vi "add-spectrum-eventSD.vi"(1 "cluster in":T1={"Kinetics"=[], "Spectrum"=[], "Experiments groups"=[], "GRAPH EXPERIMENTAL DATA"=[], "error out"={"status"=FALSE, "code"=0, "source"=""}, "group"=0, "exp selected"=0, "# exp"=0, "kinetics plot names"=[], "spectra plot names"=[], "FromToWave"={"FromWave"=0.0, "ToWave"=0.0}, "Laser shutter task"="", "Accelerator task"="", "Motor task"="", "GRAPH EXPERIMENTAL DATA ref"=refnum, "timedelays"=[0.0, 0.0, 0.0, 0.0, 0.0, 0.0, 0.0, 0.06019061100911815, 0.0521779104562645, 0.045231877429679615, 0.03921051490799832, 0.033990728811568754, 0.029465811603150715, 0.025543260876973825, 0.02214288834180205, 0.01919518054014414, 0.016639877791965713, 0.014424742312398925, 0.012504490320209958, 0.010839866306230088, 0.009396840537117498, 0.008145913389103785, 0.00706151229029317, 0.006121468943269439, 0.005306566140927374, 0.004600144911132549, 0.003987763959109073, 0.0034569044455719407, 0.00299671406541447, 0.0025977851951783253, 0.0022519625739982996, 0.00195217658646366, 0.0016922987392150965, 0.0014670163768006634, 0.0012717240756200802, 0.0011024294957352762, 0.0009556717658856477, 0.0008284507332614981, 0.0007181656316962257, 0.0006225619144775864, 0.0005396851648867825, 0.00046784114226338394, 0.0004055611468220084, 0.0003515719951773376, 0.00030476999279031153, 0.00026419837125694315, 0.00022902772919263772, 0.0001985390768670671, 0.0001721091379728629, 0.00014919760805372974, 0.00012933610911736794], "wavelengths"=[0.0, 0.0, 0.0, 0.0, 0.0, 0.0, 0.0, 0.06019061100911815, 0.0521779104562645, 0.045231877429679615, 0.03921051490799832, 0.033990728811568754, 0.029465811603150715, 0.025543260876973825, 0.02214288834180205, 0.01919518054014414, 0.016639877791965713, 0.014424742312398925, 0.012504490320209958, 0.010839866306230088, 0.009396840537117498, 0.008145913389103785, 0.00706151229029317, 0.006121468943269439, 0.005306566140927374, 0.004600144911132549, 0.003987763959109073, 0.0034569044455719407, 0.00299671406541447, 0.0025977851951783253, 0.0022519625739982996, 0.00195217658646366, 0.0016922987392150965, 0.0014670163768006634, 0.0012717240756200802, 0.0011024294957352762, 0.0009556717658856477, 0.0008284507332614981, 0.0007181656316962257, 0.0006225619144775864, 0.0005396851648867825, 0.00046784114226338394, 0.0004055611468220084, 0.0003515719951773376, 0.00030476999279031153, 0.00026419837125694315, 0.00022902772919263772, 0.0001985390768670671, 0.0001721091379728629, 0.00014919760805372974, 0.00012933610911736794], "Experiment"=refnum, "Commentaires exp"=refnum, "FromToDelay"={"FromDelay"=0.0, "ToDelay"=0.0}}, 2 "redraw event":refnum<user-event>) -> (0 "cluster out":T1={"Kinetics"=[], "Spectrum"=[], "Experiments groups"=[], "GRAPH EXPERIMENTAL DATA"=[], "error out"={"status"=FALSE, "code"=0, "source"=""}, "group"=0, "exp selected"=0, "# exp"=0, "kinetics plot names"=[], "spectra plot names"=[], "FromToWave"={"FromWave"=0.0, "ToWave"=0.0}, "Laser shutter task"="", "Accelerator task"="", "Motor task"="", "GRAPH EXPERIMENTAL DATA ref"=refnum, "timedelays"=[0.0, 0.0, 0.0, 0.0, 0.0, 0.0, 0.0, 0.06019061100911815, 0.0521779104562645, 0.045231877429679615, 0.03921051490799832, 0.033990728811568754, 0.029465811603150715, 0.025543260876973825, 0.02214288834180205, 0.01919518054014414, 0.016639877791965713, 0.014424742312398925, 0.012504490320209958, 0.010839866306230088, 0.009396840537117498, 0.008145913389103785, 0.00706151229029317, 0.006121468943269439, 0.005306566140927374, 0.004600144911132549, 0.003987763959109073, 0.0034569044455719407, 0.00299671406541447, 0.0025977851951783253, 0.0022519625739982996, 0.00195217658646366, 0.0016922987392150965, 0.0014670163768006634, 0.0012717240756200802, 0.0011024294957352762, 0.0009556717658856477, 0.0008284507332614981, 0.0007181656316962257, 0.0006225619144775864, 0.0005396851648867825, 0.00046784114226338394, 0.0004055611468220084, 0.0003515719951773376, 0.00030476999279031153, 0.00026419837125694315, 0.00022902772919263772, 0.0001985390768670671, 0.0001721091379728629, 0.00014919760805372974, 0.00012933610911736794], "wavelengths"=[0.0, 0.0, 0.0, 0.0, 0.0, 0.0, 0.0, 0.06019061100911815, 0.0521779104562645, 0.045231877429679615, 0.03921051490799832, 0.033990728811568754, 0.029465811603150715, 0.025543260876973825, 0.02214288834180205, 0.01919518054014414, 0.016639877791965713, 0.014424742312398925, 0.012504490320209958, 0.010839866306230088, 0.009396840537117498, 0.008145913389103785, 0.00706151229029317, 0.006121468943269439, 0.005306566140927374, 0.004600144911132549, 0.003987763959109073, 0.0034569044455719407, 0.00299671406541447, 0.0025977851951783253, 0.0022519625739982996, 0.00195217658646366, 0.0016922987392150965, 0.0014670163768006634, 0.0012717240756200802, 0.0011024294957352762, 0.0009556717658856477, 0.0008284507332614981, 0.0007181656316962257, 0.0006225619144775864, 0.0005396851648867825, 0.00046784114226338394, 0.0004055611468220084, 0.0003515719951773376, 0.00030476999279031153, 0.00026419837125694315, 0.00022902772919263772, 0.0001985390768670671, 0.0001721091379728629, 0.00014919760805372974, 0.00012933610911736794], "Experiment"=refnum, "Commentaires exp"=refnum, "FromToDelay"={"FromDelay"=0.0, "ToDelay"=0.0}})   [LabVIEW 2015]
uses:
  controls/control-cluster.ctl
  Classes/Experiments_group.lvclass
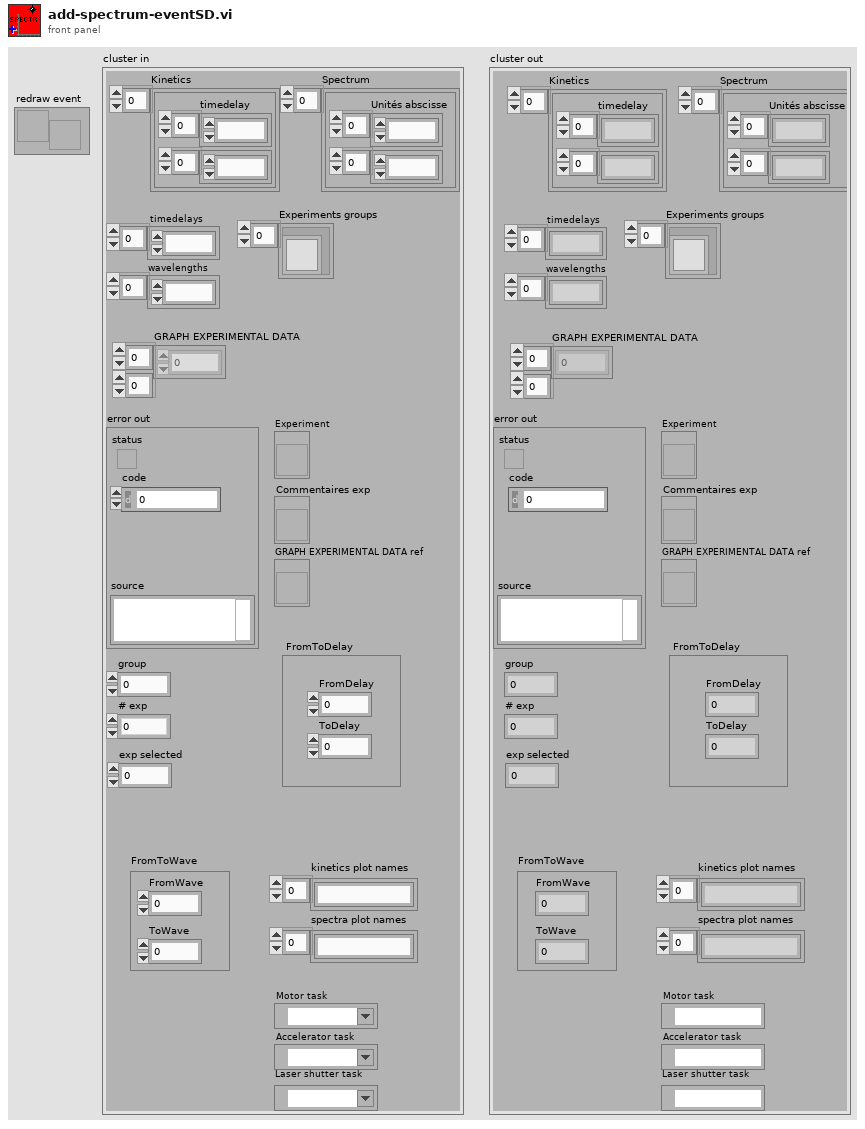
[diagram p1: front panel]
types:
  T1 = typedef "control-cluster.ctl" = cluster{"Kinetics":cluster{"timedelay":dbl[], dbl[]}[], "Spectrum":cluster{"Unités abscisse":dbl[], dbl[]}[], "Experiments groups":refnum<class "Experiments_group.lvclass">[], "GRAPH EXPERIMENTAL DATA":dbl[][], "error out":errorcluster, "group":i32, "exp selected":i32, "# exp":i32, "kinetics plot names":string[], "spectra plot names":string[], "FromToWave":cluster{"FromWave":dbl, "ToWave":dbl}, "Laser shutter task":refnum<k21>, "Accelerator task":refnum<k21>, "Motor task":refnum<k21>, "GRAPH EXPERIMENTAL DATA ref":refnum<vi>, "timedelays":dbl[], "wavelengths":dbl[], "Experiment":refnum<vi>, "Commentaires exp":refnum<vi>, "FromToDelay":cluster{"FromDelay":dbl, "ToDelay":dbl}}
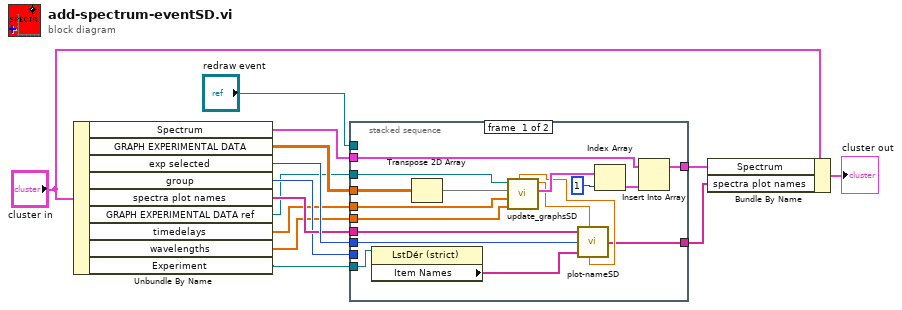
[diagram p0: block diagram]
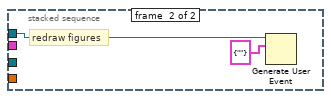
[diagram p2: hidden frame]
diagram:
  n1 = Unbundle By Name("cluster in") -> ("Spectrum"=w11:cluster{"Unités abscisse":dbl[], dbl[]}[], "GRAPH EXPERIMENTAL DATA"=w9:dbl[][], "exp selected"=w8:i32, "group"=w5:i32, "spectra plot names"=w6:string[], "GRAPH EXPERIMENTAL DATA ref"=w4:refnum<vi>, "timedelays"=w3:dbl[], "wavelengths"=w2:dbl[], "Experiment"=w1:refnum<vi>)
  n2 = stacked-sequence {
    tunnel: [w27 _] -> w10
    tunnel: "redraw event" -> [_ w32]
    tunnel: w11 -> [w23 _]
    tunnel: w9 -> [w22 _]
    tunnel: w8 -> [w18 _]
    tunnel: [w21 _] -> w7
    tunnel: w6 -> [w20 _]
    tunnel: w1 -> [w19 _]
    tunnel: w5 -> [_ _]
    tunnel: w4 -> [w17 _]
    tunnel: w3 -> [w16 _]
    tunnel: w2 -> [w15 _]
    frame #0 {
      n3 = property on="Property Node" class="LstDér (strict)"(reference=w19) -> ("Item Names"=w24:string[])  [unwired: 1 in, 2 out]
      n4 = Transpose 2D Array(2D array=w22) -> (transposed array=w31:dbl[][])
      n5 = call "update_graphsSD.vi"("wavelengths"=w15, "timedelays"=w16, "data"=w31, "IntensityGraph in"=w17) -> ("Spectrum"=w30:cluster{"Unités abscisse":dbl[], dbl[]}[], "To time"=w25:dbl, "From  time"=w26:dbl)  [unwired: 3 out]
      n6 = call "plot-nameSD.vi"("plot names in"=w20, "To"=w25, "exp selected"=w18, "Item Names"=w24, "from"=w26) -> ("plot names out"=w21:string[])
      n7 = Index Array(array=w30, index=1) -> (element=w29:cluster{"Unités abscisse":dbl[], dbl[]})
      n8 = Insert Into Array(array=w23, new element=w29) -> (w27:cluster{"Unités abscisse":dbl[], dbl[]}[])  [unwired: 1 in]
    }
    frame #1 {
      # "redraw figures"
      n9 = Generate User Event(user event=w32, event data cluster=cluster{"what to redraw":string} {"what to redraw"=""} ("event data")) -> ()  [unwired: 2 in, 2 out]
    }
  }
  n10 = Bundle By Name(cluster="cluster in", "Spectrum"=w10, "spectra plot names"=w7) -> (→"cluster out":T1)
